vi "python hdf5 simulate multiple scans.vi"() -> ()   [LabVIEW 2020]
panel:
  in  "# scans":i32
  out "x-y":u32
  out "data string":string
  out "return value 2":T1
  out "error out":errorcluster
  out "open error":string
  in  "hdf5 root path":path=path "C:/GEECS/data"
  in  "# shots in scan":i32=1
  out "time per image (ms)":dbl=1.0
  out "write image time (ms)":u32=1
  out "open session  and open_writetime":u32=368
  in  "camera name":string="Camera1"
  in  "Python version":string="3.8"
  in  "module path":path=path "C:/GEECS/Developers Version/source/Axel/openPMD-CCD/openpmd_ccd_labview.py"
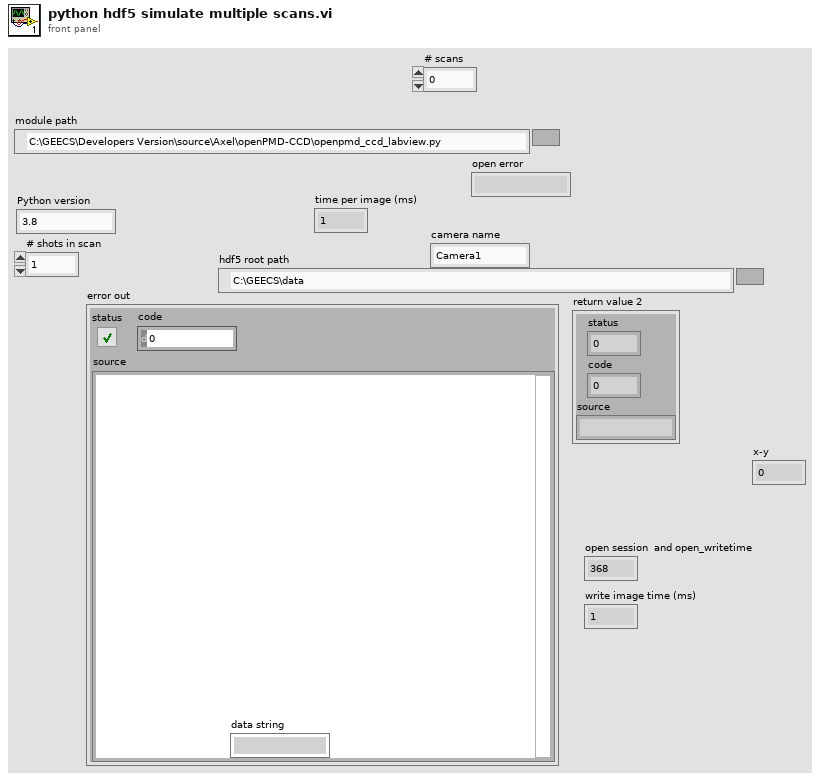
[diagram p1: front panel]
types:
  T1 = cluster{"status":i32, "code":i32, "source":string}
  T2 = enum32{"Map Pixel Pointer", "Unmap Pixel Pointer", "Get Pixels Infos"}
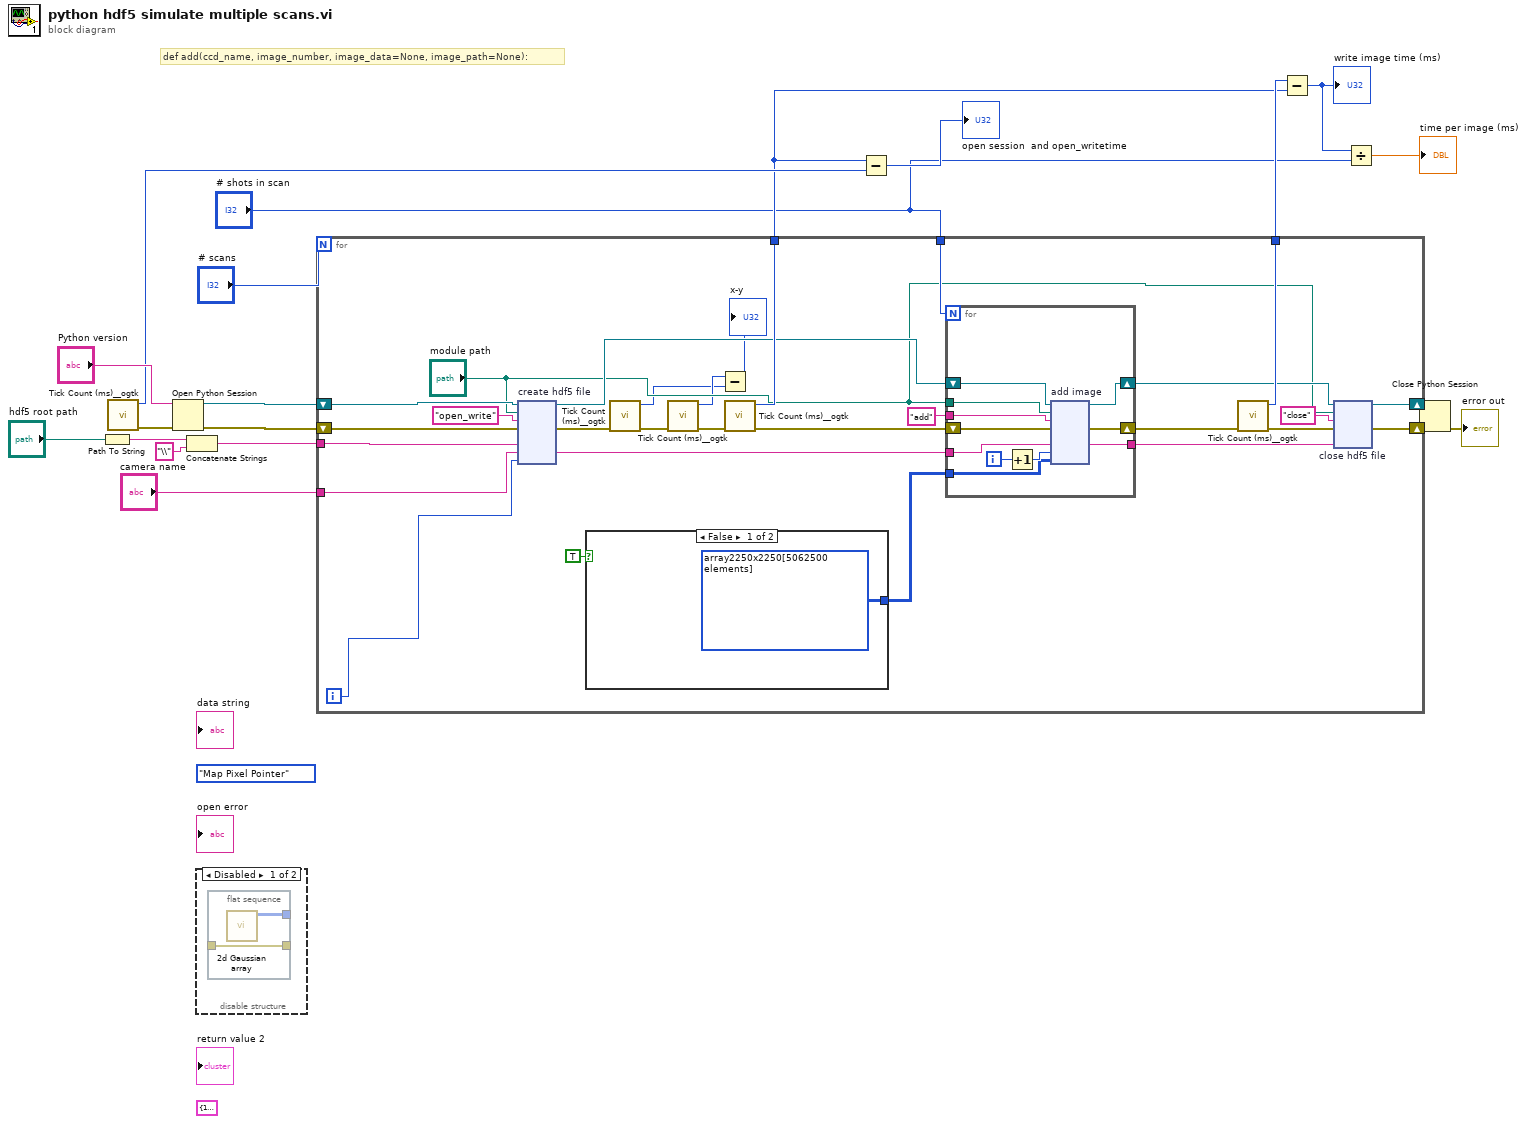
[diagram p0: block diagram]
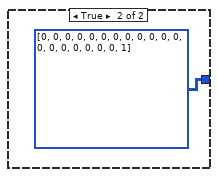
[diagram p2: hidden frame]
diagram:
  (unwired) T2."Map Pixel Pointer" ("Function")
  (unwired) T1 {"status"=1, "code"=1, "source"=""}
  # "def add(ccd_name, image_number, image_data=None, image_path=None):"
  n1 = Path To String(path="hdf5 root path") -> (string=w8:string)
  n2 = call <userlib>:"Tick Count (ms)__ogtk.vi"() -> ("error out"=w18:errorcluster, "millisecond timer value"=w19:u32)  [unwired: 10 in]
  n3 = Open Python Session(python version="Python version", 3:w18) -> (session out=w14:refnum<k35>, error out=w4:errorcluster)  [unwired: 1 in]
  n4 = Concatenate Strings(w8, "\\") -> (w6:string)
  n5 = disable-structure shown="Disabled" {
    frame Disabled {
      n6 = flat-sequence {
        tunnel: [w22] -> _
        tunnel: _ -> [w21]
        tunnel: [w21] -> _
        frame #0 {
          n7 = call "2d Gaussian array.vi"() -> ("Intensity Graph"=w22:u16[][])  [unwired: 11 in]
        }
      }
    }
    frame Enabled {
    }
  }
  n8 = for {
    N: "# scans" -> [_]
    tunnel: [w49] -> w17
    tunnel: [w48] -> w16
    tunnel: "# shots in scan" -> [w45]
    tunnel: w6 -> [w40]
    tunnel: "camera name" -> [w33]
    shift-right: [w41] -> w10
    shift-left: w14 -> [w47]
    shift-right: [w37] -> w5
    shift-left: w4 -> [w34]
    i -> [w23]
    n9 = node "create hdf5 file"(w47, "module path", "open_write" ("open h5 function"), w34, w40, w33, w23) -> (w46:refnum<k35>, w27:errorcluster, w39:string)  [unwired: 4 in, 2 out]
    n10 = case shown="False" TRUE ("small image") {
      tunnel: [u16[][] array2250x2250[5062500 elements] ("Array") u16[][] [[0, 0, 0, 0, 0], [0, 0, 0, 0, 0], [0, 0, 0, 0, 0], [0, 0, 0, 0, 1]]] -> w25
      frame False {
      }
      frame True {
      }
    }
    n11 = call <userlib>:"Tick Count (ms)__ogtk.vi"("error in (no error)"=w27) -> ("error out"=w24:errorcluster, "millisecond timer value"=w29:u32)  [unwired: 9 in]
    n12 = call <userlib>:"Tick Count (ms)__ogtk.vi"("error in (no error)"=w24) -> ("error out"=w26:errorcluster, "millisecond timer value"=w30:u32)  [unwired: 9 in]
    n13 = Subtract(x=w30, y=w29) -> (x-y=→"x-y":u32)
    n14 = call <userlib>:"Tick Count (ms)__ogtk.vi"("error in (no error)"=w26) -> ("error out"=w50:errorcluster, "millisecond timer value"=w48:u32)  [unwired: 9 in]
    n15 = for {
      N: w45 -> [_]
      tunnel: "module path" -> [w62]
      tunnel: "add" ("function name") -> [w54]
      tunnel: w39 -> [w57]
      shift-right: [w63] -> w44
      shift-left: w46 -> [w64]
      shift-right: [w60] -> w35
      shift-left: w50 -> [w61]
      tunnel: [w59] -> w38
      tunnel: w25 -> [w55]
      i -> [w58]
      n16 = Increment(x=w58) -> (x+1=w56:i32)
      n17 = node "add image"(w64, w62, w54, w61, w57, w56, w55) -> (w63:refnum<k35>, w60:errorcluster, w59:string)  [unwired: 4 in, 2 out]
    }
    n18 = call <userlib>:"Tick Count (ms)__ogtk.vi"("error in (no error)"=w35) -> ("error out"=w36:errorcluster, "millisecond timer value"=w49:u32)  [unwired: 9 in]
    n19 = node "close hdf5 file"(w44, "module path", "close" ("function name"), w36, w38) -> (w41:refnum<k35>, w37:errorcluster)  [unwired: 3 in, 2 out]
  }
  n20 = Subtract(x=w16, y=w19) -> (x-y=→"open session  and open_writetime":u32)
  n21 = Subtract(x=w17, y=w16) -> (x-y=w13:u32)
  "write image time (ms)" <- w13
  n22 = Divide(x=w13, y="# shots in scan") -> (x/y=→"time per image (ms)":dbl)
  n23 = Close Python Session(session in=w10, error in=w5) -> (11:→"error out":errorcluster)
